vi "Get Target Name.vi"(8 "error in (no error)":errorcluster, 11 "Node Ptr":T1 format="%.0x") -> (0 "error out":errorcluster, 1 "found":bool, 2 "target name":string, 3 "Item Ref out":T1 format="%.0x")   [LabVIEW 2021, in "DSF System Explorer.lvlib"]
uses:
  DSF System Explorer.lvlib
  <vilib>/NI VeriStand/Custom Device API/Custom Device Item Ref.ctl
  <vilib>/NI VeriStand/Custom Device API/Custom Device API.lvlib
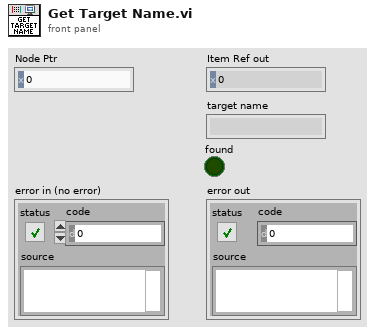
[diagram p1: front panel]
types:
  T1 = typedef "Custom Device API.lvlib/Custom Device Item Ref.ctl" = u64
  T2 = typedef "Custom Device API.lvlib/Custom Device Item Info.ctl" = cluster{"Name":string, "Is Channel":bool, "GUID":string, "Is Waveform":bool}
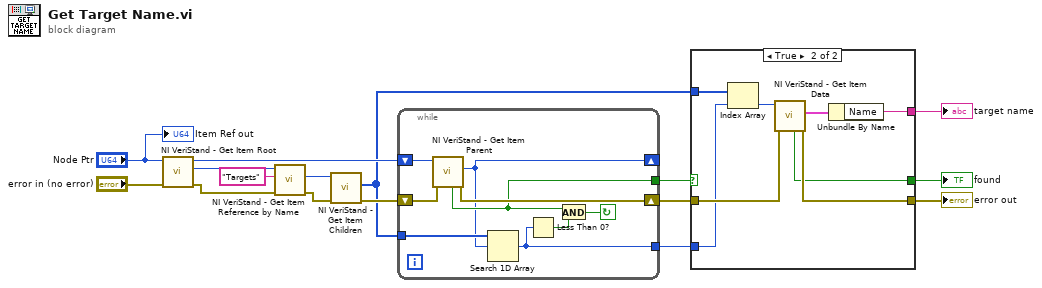
[diagram p0: block diagram]
diagram:
  n1 = call <vilib>:"NI VeriStand - Get Item Root.vi"("error in (no error)"="error in (no error)", "Item Ref in"="Node Ptr") -> ("error out"=w12:errorcluster, "Root Ref out"=w16:T1, "Item Ref out"=w9:T1)  [unwired: 6 in, 1 out]
  n2 = call <vilib>:"NI VeriStand - Get Item Reference by Name.vi"("error in (no error)"=w12, "Item Name"="Targets", "Parent Ref in"=w16) -> ("error out"=w11:errorcluster, "Item Ref"=w14:T1)  [unwired: 5 in, 2 out]
  n3 = call <vilib>:"NI VeriStand - Get Item Children.vi"("error in (no error)"=w11, "Item Ref in"=w14) -> ("error out"=w10:errorcluster, "Child Refs"=w5:T1[])  [unwired: 6 in, 2 out]
  n4 = while {
    shift-right: [w18] -> _
    shift-left: w9 -> [w25]
    shift-right: [w23] -> w7
    shift-left: w10 -> [w24]
    tunnel: w5 -> [w22]
    tunnel: [w19] -> w6
    tunnel: [w17] -> w4
    stop <- w20 continue-if-true
    n5 = call <vilib>:"NI VeriStand - Get Item Parent.vi"("error in (no error)"=w24, "Item Ref in"=w25) -> ("error out"=w23:errorcluster, "Parent Ref"=w18:T1, "Found"=w19:bool)  [unwired: 6 in, 1 out]
    n6 = Search 1D Array(1D array=w22, element=w18) -> (index of element=w17:i32)  [unwired: 1 in]
    n7 = Less Than 0?(x=w17) -> (x < 0?=w21:bool)
    n8 = And(x=w19, y=w21) -> (x .and. y?=w20:bool)
  }
  n9 = case shown="True" w6 {
    selector: w6 -> [w26 _]
    tunnel: w7 -> [w27 w33]
    tunnel: w5 -> [_ w35]
    tunnel: w4 -> [_ w31]
    tunnel: [w27 w32] -> w3
    tunnel: [_ w29] -> w2
    tunnel: [w26 w28] -> w1
    frame False {
    }
    frame True {
      n10 = Index Array(array=w35, index=w31) -> (element=w34:T1)
      n11 = call <vilib>:"NI VeriStand - Get Item Data.vi"("error in (no error)"=w33, "Item Ref in"=w34) -> ("error out"=w32:errorcluster, "Item Info"=w30:T2, "Found"=w28:bool)  [unwired: 6 in, 1 out]
      n12 = Unbundle By Name(w30) -> ("Name"=w29:string)
    }
  }
  "error out" <- w3
  "target name" <- w2
  "found" <- w1
  "Item Ref out" <- "Node Ptr"
